vi "Get Thermostat Mode.vi"(7 "Use Cached Data?":bool, 8 "Error In":errorcluster, 10 "Device Name":string, 11 "Nest Config":T2) -> (0 "Error Out":errorcluster, 2 "Thermostat Mode":T1, 3 "Nest Config":T2)   [LabVIEW 2013, in "LVH-Nest.lvlib"]
doc: "Read the mode of the specified Nest device (heat, cool, heat/cool)."
uses:
  LVH-Nest.lvlib
  Private/Type Defs/Nest Config.ctl
  <vilib>/httpClient/ClientHandle.ctl
  Private/Type Defs/Session Data.ctl
  Private/Type Defs/Thermostat Mode.ctl
  <vilib>/httpClient/LabVIEWHTTPClient.lvlib
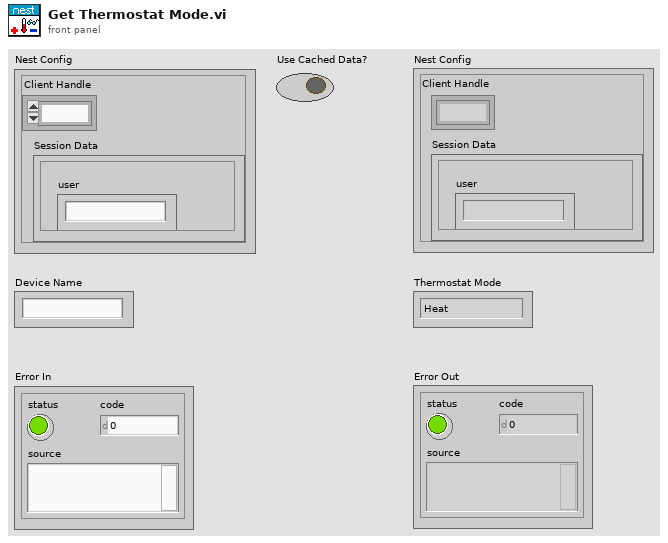
[diagram p1: front panel]
types:
  T1 = typedef "LVH-Nest.lvlib/Thermostat Mode.ctl" = enum16{"Heat", "Cool", "Heat / Cool"}
  T2 = typedef "LVH-Nest.lvlib/Nest Config.ctl" = cluster{"Client Handle":T3, "Session Data":T4}
  T3 = typedef "LabVIEWHTTPClient.lvlib/ClientHandle.ctl" = refnum<k1>
  T4 = typedef "LVH-Nest.lvlib/Session Data.ctl" = cluster{"is_superuser":bool, "is_staff":bool, "urls":cluster{"transport_url":string, "rubyapi_url":string, "weather_url":string, "log_upload_url":string, "support_url":string}, "limits":cluster{"thermostats_per_structure":u32, "structures":u32, "thermostats":u32, "smoke_detectors":u32, "smoke_detectors_per_structure":u32}, "access_token":string, "userid":string, "expires_in":string, "email":string, "user":string, "language":string}
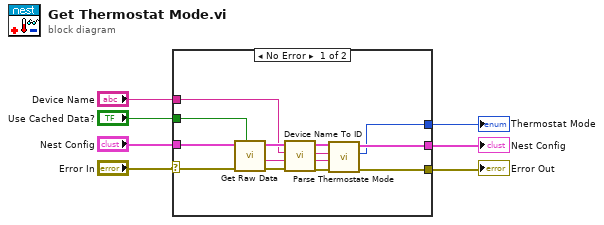
[diagram p0: block diagram]
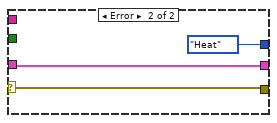
[diagram p2: hidden frame]
diagram:
  n1 = case shown="No Error" "Error In" {
    selector: "Error In" -> [w15 w24]
    tunnel: "Use Cached Data?" -> [w21 _]
    tunnel: "Nest Config" -> [w20 w23]
    tunnel: "Device Name" -> [w18 _]
    tunnel: [w10 w24] -> w4
    tunnel: [w9 w23] -> w3
    tunnel: [w8 Thermostat_Mode."Heat" ("Thermostat Mode")] -> w1
    frame No Error {
      n2 = call "Get Raw Data.vi"("Use Cached Data?"=w21, "Error In"=w15, "Nest Config"=w20) -> ("Error Out"=w17:errorcluster, "Data"=w16:string, "Nest Config"=w19:T2)  [unwired: 6 in]
      n3 = call "Device Name To ID.vi"("Error In"=w17, "Data"=w16, "Device Name"=w18, "Nest Config"=w19) -> ("Error Out"=w11:errorcluster, "Data"=w12:string, "Device ID"=w13:string, "Nest Config"=w14:T2)  [unwired: 4 in]
      n4 = call "Parse Thermostate Mode.vi"("Error In"=w11, "Data"=w12, "Device ID"=w13, "Nest Config"=w14) -> ("Error Out"=w10:errorcluster, "Thermostat Mode"=w8:T1, "Nest Config"=w9:T2)  [unwired: 4 in, 1 out]
    }
    frame Error {
    }
  }
  "Error Out" <- w4
  "Nest Config" <- w3
  "Thermostat Mode" <- w1
